vi "Storage Data.vi"(8 "Error In":errorcluster, 9 "Time Out In ms":i32=-1, 10 "Data In":variant, 11 "Circular Buffer 2D U16 DVR Queue Circular Buffer in":refnum<class "Circular Buffer 2D U16 DVR Queue Circular Buffer.lvclass">) -> (0 "Error Out":errorcluster, 1 "Time Out":bool, 3 "Circular Buffer 2D U16 DVR Queue Circular Buffer out":refnum<class "Circular Buffer 2D U16 DVR Queue Circular Buffer.lvclass">)   [LabVIEW 2024, in "Circular Buffer 2D U16 DVR Queue Circular Buffer.lvclass"]
uses:
  Circular Buffer 2D U16 DVR Queue Circular Buffer.lvclass
  Circular Buffer 2D U16 DVR Queue Circular Buffer.lvclass/Circular Buffer 2D U16 DVR Queue Circular Buffer.ctl
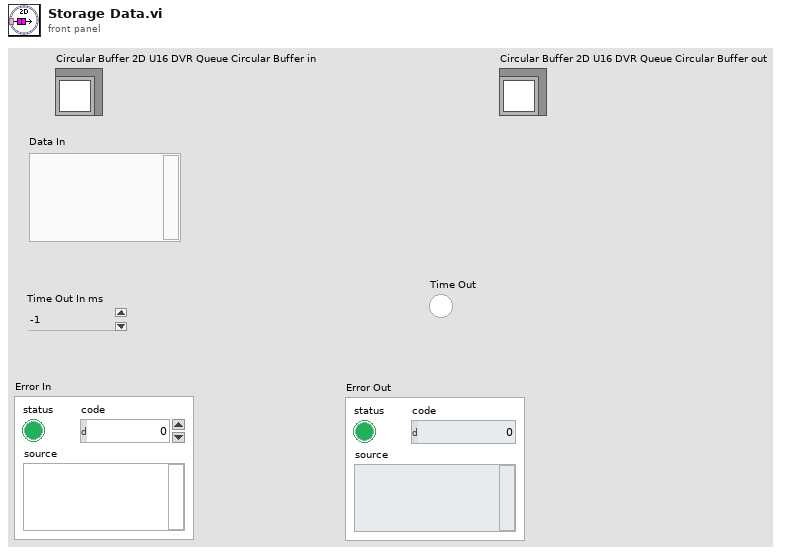
[diagram p1: front panel]
types:
  T1 = typedef "2D U16 DVR Queue.ctl" = refnum<queue>
  T2 = typedef "2D U16 DVR.ctl" = refnum<data-value>
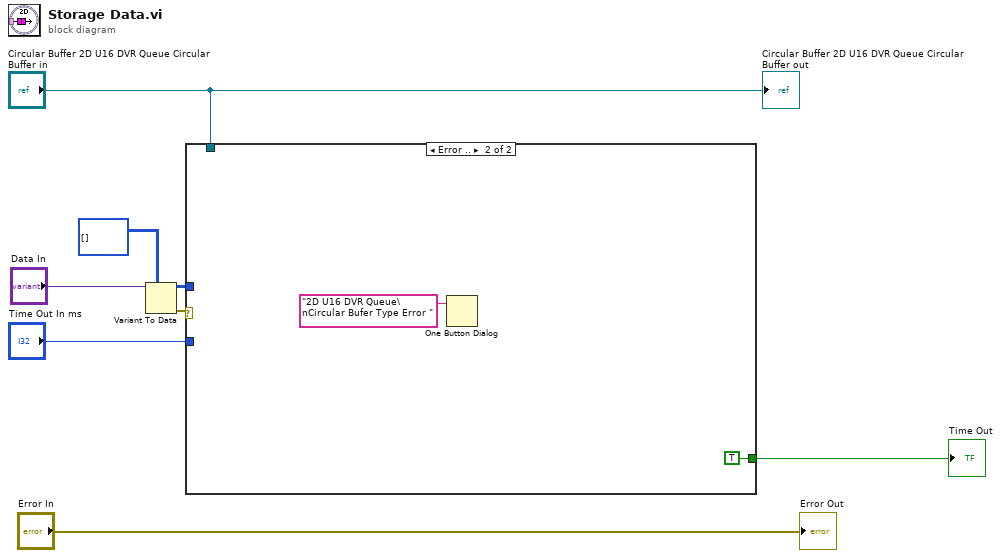
[diagram p0: block diagram]
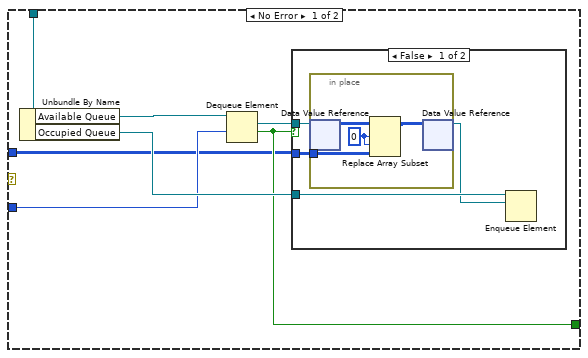
[diagram p2: hidden frame]
diagram:
  n1 = Variant To Data(type=u16[][] [] ("Data In"), Variant="Data In") -> (data=w3:u16[][], error out=w2:errorcluster)  [unwired: 1 in]
  n2 = case shown="Error .." w2 {
    tunnel: "Time Out In ms" -> [w13 _]
    tunnel: [w11 TRUE ("timed out?")] -> w7
    tunnel: "Circular Buffer 2D U16 DVR Queue Circular Buffer in" -> [w10 _]
    tunnel: w3 -> [w9 _]
    frame No Error {
      n3 = Unbundle By Name(w10) -> ("Available Queue"=w14:T1, "Occupied Queue"=w15:T1)
      n4 = Dequeue Element(queue=w14, timeout in ms (-1)=w13) -> (element=w12:T2, timed out?=w11:bool)  [unwired: 1 in, 2 out]
      n5 = case shown="False" w11 {
        tunnel: w12 -> [w19 _]
        tunnel: w15 -> [w18 _]
        tunnel: w9 -> [w16 _]
        frame False {
          n6 = in-place {
            in-place-border: w16 -> [w20]
            w21 = 0 ("index (row)")
            n7 = in-place-dvr #1(w19) -> (w23:u16[][])  [unwired: 1 out]
            n8 = Replace Array Subset(array=w23, new element=w20, index (row)=w21, index (col)=w21) -> (w22:u16[][])
            n9 = in-place-dvr #1(w22) -> (w17:T2)  [unwired: 1 out]
          }
          n10 = Enqueue Element(queue=w18, element=w17) -> ()  [unwired: 2 in, 3 out]
        }
        frame True {
        }
      }
    }
    frame Error {
      n11 = One Button Dialog(message="2D U16 DVR Queue\nCircular Bufer Type Error ") -> ()  [unwired: 1 in, 1 out]
    }
  }
  "Time Out" <- w7
  "Circular Buffer 2D U16 DVR Queue Circular Buffer out" <- "Circular Buffer 2D U16 DVR Queue Circular Buffer in"
  "Error Out" <- "Error In"
